vi "19-Rotate.vi"(4 "Rotate By":dbl, 5 "Number of Rotations":i32, 6 "Initial Rotation":dbl, 7 "Rotation Axis":enum16{"x", "y", "z"}(ring), 11 "Sensor":cluster{"Name":string, "Beacons":i32[][]}) -> (3 "Sensor Rotations":cluster{"Name":string, "Beacons":i32[][]}[](array[cluster]))   [LabVIEW 2019, in "19.lvlib"]
uses:
  19.lvlib
  <vilib>/Analysis/coordinate.llb/2D Cartesian Coordinate Rotation (Array).vi
  <vilib>/Analysis/NI_AALPro.lvlib
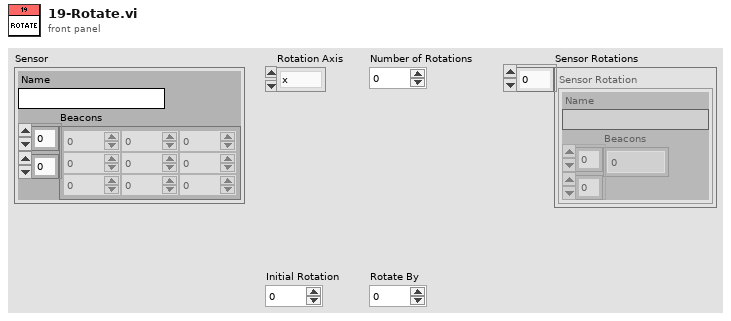
[diagram p1: front panel]
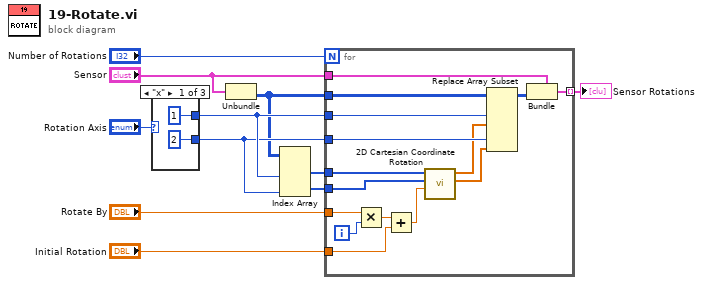
[diagram p0: block diagram]
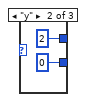
[diagram p2: hidden frame]
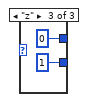
[diagram p3: hidden frame]
diagram:
  n1 = case shown="\"x\"" "Rotation Axis" {
    tunnel: [1 ("disabled index (col)") 2 ("disabled index (col)") 0 ("disabled index (col)")] -> w4
    tunnel: [2 ("index (col)") 0 ("index (col)") 1 ("index (col)")] -> w3
    frame "x" {
    }
    frame "y" {
    }
    frame "z" {
    }
  }
  n2 = Unbundle("Sensor") -> ("Beacons"=w1:i32[][])  [unwired: 1 out]
  n3 = Index Array(array=w1, index (col) #1=w4, index (col) #2=w3) -> (element #1=w9:i32[], element #2=w10:i32[])  [unwired: 2 in]
  n4 = for {
    N: "Number of Rotations" -> [_]
    tunnel: "Rotate By" -> [w29]
    tunnel: w9 -> [w32]
    tunnel: w10 -> [w31]
    tunnel: [w18] -> w7 mode=indexing
    tunnel: "Sensor" -> [w28]
    tunnel: w1 -> [w27]
    tunnel: w4 -> [w26]
    tunnel: w3 -> [w25]
    tunnel: "Initial Rotation" -> [w19]
    i -> [w21]
    n5 = Multiply(x=w29, y=w21) -> (x*y=w30:dbl)
    n6 = Add(x=w30, y=w19) -> (x+y=w20:dbl)
    n7 = call-poly <vilib>:"2D Cartesian Coordinate Rotation.vi"("theta"=w20, "Y"=w31, "X"=w32) -> ("Y Out"=w23:dbl[], "X Out"=w24:dbl[])  [unwired: 6 in, 1 out]
    n8 = Replace Array Subset(array=w27, new element #1=w24, index (col) #1=w26, new element #2=w23, index (col) #2=w25) -> (w22:i32[][])  [unwired: 2 in]
    n9 = Bundle(cluster=w28, "Beacons"=w22) -> (w18:cluster{"Name":string, "Beacons":i32[][]})  [unwired: 1 in]
  }
  "Sensor Rotations" <- w7
